vi "save-device.vi"(6 "Proc Name":string, 9 "Module Name":string, 10 "Base Folder":string, 11 "Device":T1 caption="Device Setup" {"Schedular"."sched-pairs"."start" format="%<%H:%M %d/%m>T"; "Schedular"."sched-pairs"."stop" format="%<%H:%M %d/%m>T"; "Timeout" min=1}) -> (0 "error out":errorcluster, 2 "procNameID":string)   [LabVIEW 2024]
uses:
  controls/controller.ctl
  controls/sched-cluster.ctl
  controls/UiScheduleTimestamp.ctl
  controls/UiDeviceSensorParams.ctl
  controls/UiDeviceSensorEquality.ctl
  controls/device-mode.ctl
  controls/UiProcHeader.ctl
panel:
  out "Procedure out":variant[](array[variant])
  # "Pulse [sec]"
  # "Period [sec]"
  # "Sensor"
  # "Scheduler"
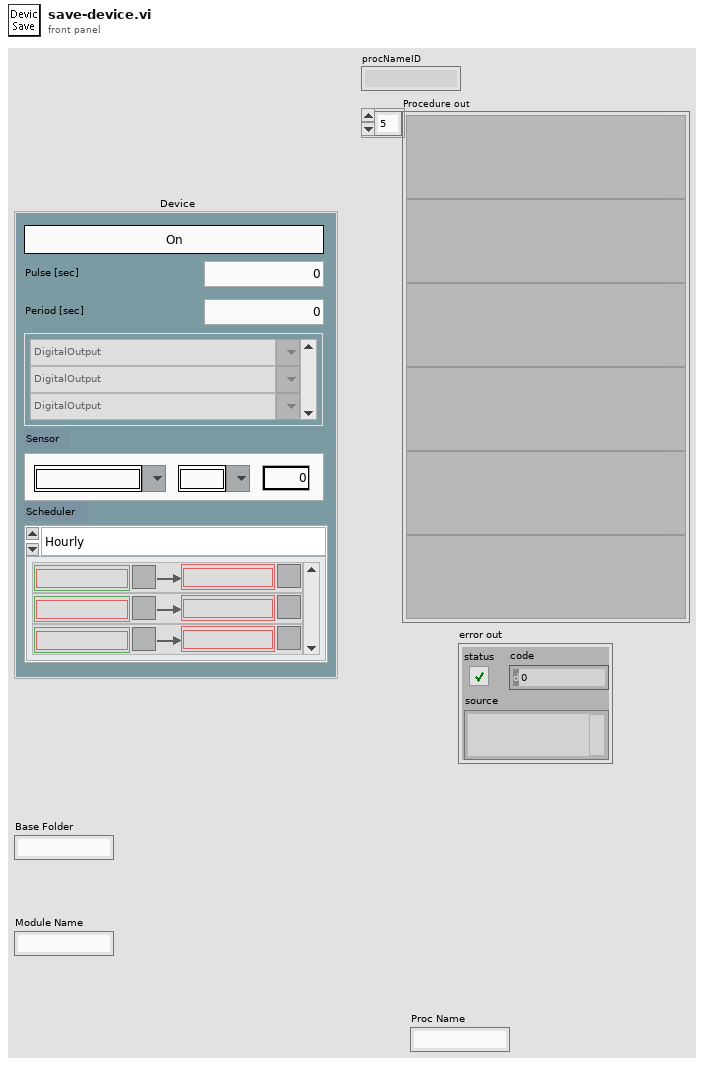
[diagram p1: front panel]
types:
  T1 = typedef "controller.ctl" = cluster{"Schedular":T2, "Sensor":T4, "Outputs":string[], "Interval":u32, "Timeout":u16, "Mode":T6}
  T2 = typedef "sched-cluster.ctl" = cluster{"sched-mode":enum16{"Hourly", "Daily", "Weekly", "Date"}, "sched-pairs":cluster{"start":T3, "stop":T3}[]}
  T3 = typedef "UiScheduleTimestamp.ctl" = timestamp
  T4 = typedef "UiDeviceSensorParams.ctl" = cluster{"Input":string, "Comparison":T5, "Setpoint":dbl}
  T5 = typedef "UiDeviceSensorEquality.ctl" = string
  T6 = typedef "device-mode.ctl" = enum16{"On", "Off", "Sense", "Sched", "Sched AND Sense", "Sched OR Sense"}
  T7 = typedef "UiProcHeader.ctl" = cluster{"Procedure Name":string, "Running":bool, "tags":string}
  T8 = typedef "UiStepBuilder.ctl" = cluster{"Step Function":T9, "ParamString":string, "Step Label":string}
  T9 = typedef "type.step-builder.ctl" = enum16{"NO_OPERATION", "DELAY-JUMP", "DELAY", "JUMP", "COMPLETE", "SCHEDULER", "IRR-CHECK", "UNIT-CHECK", "UNIT-SAMPLE", "UNIT-DOSE", "LOG-REPORT", "LOG-MESSAGE", "IO-READ", "IO-READ-MANY", "IO-WRITE", "IO-COMPARE-OUT", "IO-COMPARE-IN", "PROC-START", "PROC-STOP", "PROC-LOAD", "PROC-IS-COMPLETED", "RECORD-MOVE", "GET-RH", "GET-UV", "GET-WD", "GET-WS", "OCS-CHECK", "OCS-RECORD"}
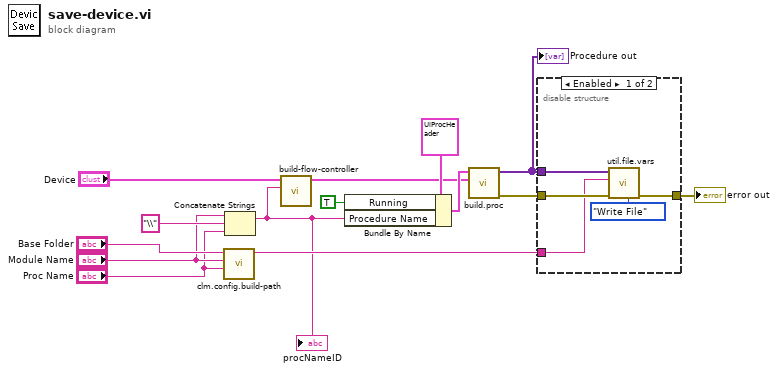
[diagram p0: block diagram]
diagram:
  n1 = call "clm.config.build-path.vi"("Proc Name"="Proc Name", "Section Name"="Module Name", "Module Name"="Base Folder") -> ("Relative Path"=w4:string)  [unwired: 8 in]
  n2 = Concatenate Strings("Module Name", "\\" ("string"), "Proc Name") -> (w1:string)
  "procNameID" <- w1
  n3 = call "build-flow-controller.vi"("Proc Name"=w1, "Device"="Device") -> ("Flow"=w5:T8[])  [unwired: 9 in]
  n4 = Bundle By Name(cluster=T7 {"Procedure Name"="MyProcExample", "Running"=TRUE, "tags"="MyProcExample"} ("Proc Head"), "Running"=TRUE, "Procedure Name"=w1) -> (w11:T7)
  n5 = call "build.proc.vi"("Flow"=w5, "Proc Head"=w11) -> ("error out"=w14:errorcluster, "Instructions"=w12:variant[])  [unwired: 8 in]
  "Procedure out" <- w12
  n6 = disable-structure shown="Enabled" {
    disable-tunnel: w14 -> [w19 w20]
    disable-tunnel: w12 -> [w18 _]
    disable-tunnel: w4 -> [w16 _]
    disable-tunnel: [w15 w20] -> w3
    frame Enabled {
      n7 = call "util.file.vars.vi"("Operation(Read)"=enum16{"Read File", "Write File"}."Write File", "error in"=w19, "Proc Name(open dialog if empty)"=w16, "Vars[] in"=w18) -> ("error out"=w15:errorcluster)  [unwired: 3 in, 4 out]
    }
    frame Disabled {
    }
  }
  "error out" <- w3
